vi "LoadData.vi"() -> (3 "Configuration Data":T1)   [LabVIEW 2014]
uses:
  Variables/Physical data.vi
  <vilib>/Utility/file.llb/Read From Spreadsheet File (string).vi
  Variables/Default global.vi
  Variables/References.vi
  <vilib>/Utility/config.llb/NI_LVConfig.lvlib
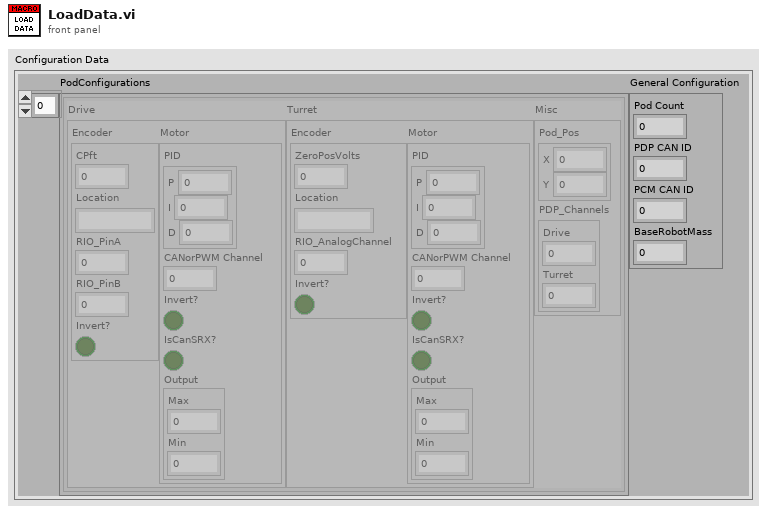
[diagram p1: front panel]
types:
  T1 = cluster{"PodConfigurations":cluster{"Drive":cluster{"Encoder":cluster{"CPft":dbl, "Location":string, "RIO_PinA":i32, "RIO_PinB":i32, "Invert?":bool}, "Motor":cluster{"PID":cluster{"P":dbl, "I":dbl, "D":dbl}, "CANorPWM Channel":i32, "Invert?":bool, "IsCanSRX?":bool, "Output":cluster{"Max":dbl, "Min":dbl}}}, "Turret":cluster{"Encoder":cluster{"ZeroPosVolts":dbl, "Location":string, "RIO_AnalogChannel":i32, "Invert?":bool}, "Motor":cluster{"PID":cluster{"P":dbl, "I":dbl, "D":dbl}, "CANorPWM Channel":i32, "Invert?":bool, "IsCanSRX?":bool, "Output":cluster{"Max":dbl, "Min":dbl}}}, "Misc":cluster{"Pod_Pos":cluster{"X":dbl, "Y":dbl}, "PDP_Channels":cluster{"Drive":i32, "Turret":i32}}}[], "General Configuration":cluster{"Pod Count":i32, "PDP CAN ID":i32, "PCM CAN ID":i32, "BaseRobotMass":dbl}}
  T2 = typedef "NI_LVConfig.lvlib/Config Data RefNum.ctl" = refnum<k1>
  T3 = enum16{"open", "replace", "create", "open or create", "replace or create", "replace or create with confirmation"}
  T4 = cluster{"String":string, "String":string, "String":string, "String":string}
  T5 = cluster{"String":dbl, "String":dbl, "String":dbl, "String":dbl}
  T6 = cluster{"String":dbl, "String":dbl, "String":dbl, "String":dbl, string}
  T7 = typedef "NI_Matrix.lvlib/RealMatrix.ctl" = dbl[][]
  T8 = cluster{"All Pod State Data":cluster{"Drive":cluster{"Drive Motor Output":dbl, "Wheel RPM":dbl, "Linear speed":dbl, "Linear acceleration":dbl, "Encoder Output":dbl, "Vmot":dbl, "Imot":dbl, "Torque":dbl, "Angular Momentum":dbl}, "Turret":cluster{"Turret Motor Output":dbl, "Turret Angle":dbl, "Turret velocity":dbl, "Turret acceleration":dbl, "Encoder Output":dbl, "Vmot":dbl, "Imot":dbl, "Torque":dbl, "Angular Momentum":dbl}, "Pod position (RCS)":cluster{"X":dbl, "Y":dbl, "Z":dbl}}[], "Global Robot Data":cluster{"Position Data":cluster{"Robot Position":cluster{"X":dbl, "Y":dbl, "Z":dbl}, "Robot Velocity":cluster{"X":dbl, "Y":dbl, "Z":dbl}, "Robot Acceleration":cluster{"X":dbl, "Y":dbl, "Z":dbl}}, "Rotation Data":cluster{"Angular Position":cluster{"X":dbl, "Y":dbl, "Z":dbl}, "Angular Velocity":cluster{"X":dbl, "Y":dbl, "Z":dbl}, "Angular Acceleration":cluster{"X":dbl, "Y":dbl, "Z":dbl}}}, "Inertial Characteristics":cluster{"Center of Mass (RCS)":cluster{"X":dbl, "Y":dbl, "Z":dbl}, "Mass Elements":cluster{"X":dbl, "Y":dbl, "Z":dbl, "Mass":dbl, "Name":string}[], "Center of Rotation (RCS)":cluster{"X":dbl, "Y":dbl, "Z":dbl}, "Tensor of Inertia":T7}}
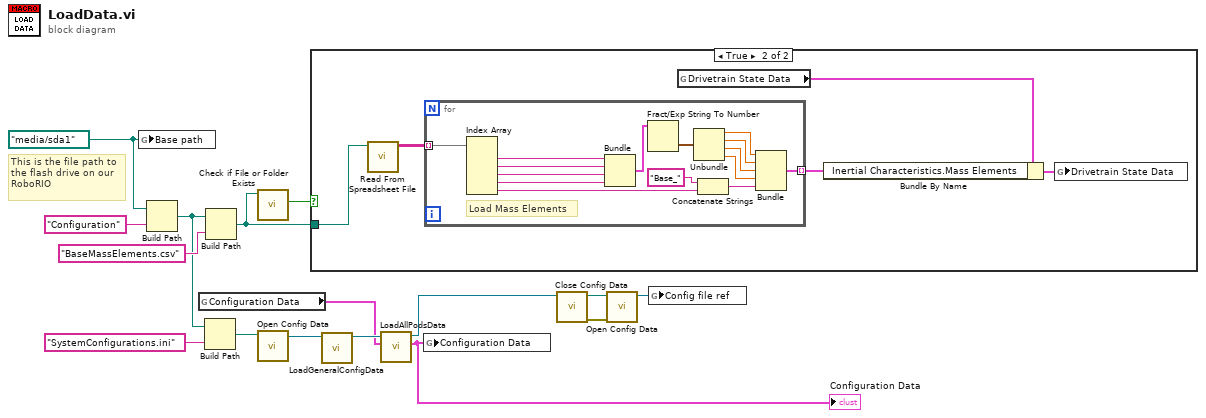
[diagram p0: block diagram]
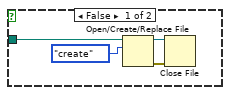
[diagram p2: hidden frame]
diagram:
  w11 = path "/media/sda1" ("Base path")
  # "This is the file path to\nthe flash drive on our\nRoboRIO"
  n1 = global write "Default global.vi" "Base path"(w11) -> ()
  n2 = Build Path(base path=w11, name or relative path="Configuration") -> (appended path=w13:path)
  n3 = global read "Physical data.vi" "Configuration Data"() -> (w2:T1)
  n4 = Build Path(base path=w13, name or relative path="SystemConfigurations.ini") -> (appended path=w12:path)
  n5 = Build Path(base path=w13, name or relative path="BaseMassElements.csv") -> (appended path=w9:path)
  n6 = call <vilib>:"Check if File or Folder Exists.vi"("path"=w9) -> ("file or folder exists?"=w10:bool)  [unwired: 8 in, 2 out]
  n7 = call <vilib>:"Open Config Data.vi"("configuration file path"=w12) -> ("refnum"=w5:T2)  [unwired: 8 in, 2 out]
  n8 = case shown="True" w10 {
    tunnel: w9 -> [w20 w21]
    frame False {
      n9 = Open/Create/Replace File(file path (use dialog)=w20, operation (0:open)=T3."create") -> (refnum out=w17:refnum<file>, error out=w18:errorcluster)  [unwired: 4 in, 1 out]
      n10 = Close File(refnum=w17, error in=w18) -> ()  [unwired: 2 out]
    }
    frame True {
      n11 = call-poly <vilib>:"Read From Spreadsheet File.vi"("file path (dialog if empty)"=w21) -> ("all rows"=w23:string[][])  [unwired: 6 in, 4 out]
      n12 = for {
        tunnel: w23 -> [w40] mode=indexing
        tunnel: [w29] -> w24 mode=indexing
        # "Load Mass Elements"
        n13 = Index Array(array=w40) -> (element #1=w38:string, element #2=w39:string, element #3=w37:string, element #4=w31:string, element #5=w27:string)  [unwired: 5 in]
        n14 = Bundle("String"=w38, "String"=w39, "String"=w37, "String"=w31) -> (w36:T4)  [unwired: 1 in]
        n15 = Fract/Exp String To Number(string=w36) -> (number=w35:T5)  [unwired: 3 in, 1 out]
        n16 = Unbundle(w35) -> ("String"=w34:dbl, "String"=w33:dbl, "String"=w32:dbl, "String"=w30:dbl)
        n17 = Concatenate Strings("Base_" ("string"), w27) -> (w26:string)
        n18 = Bundle("String"=w34, "String"=w33, "String"=w32, "String"=w30, w26) -> (w29:T6)  [unwired: 1 in]
      }
      n19 = global read "Physical data.vi" "Drivetrain State Data"() -> (w22:T8)
      n20 = Bundle By Name(cluster=w22, "Inertial Characteristics.Mass Elements"=w24) -> (w25:T8)
      n21 = global write "Physical data.vi" "Drivetrain State Data"(w25) -> ()
    }
  }
  n22 = call "LoadGeneralConfigData.vi"("Refnum in"=w5) -> ("Refnum out"=w4:T2)  [unwired: 10 in]
  n23 = call "LoadAllPodsData.vi"("Configuration Data in"=w2, "Config file Refnum in"=w4) -> ("Configuration Data out"=w1:T1, "Config fileRefnum out"=w3:T2)  [unwired: 8 in]
  "Configuration Data" <- w1
  n24 = global write "Physical data.vi" "Configuration Data"(w1) -> ()
  n25 = call <vilib>:"Close Config Data.vi"("refnum"=w3) -> ("error out"=w8:errorcluster, "file path"=w7:path)  [unwired: 9 in]
  n26 = call <vilib>:"Open Config Data.vi"("error in (no error)"=w8, "configuration file path"=w7) -> ("refnum"=w6:T2)  [unwired: 7 in, 2 out]
  n27 = global write "References.vi" "Config file ref"(w6) -> ()
